vi "write_tag_status.vi"(5 "Inicio pasada":timestamp=timestamp(3789638435.424 s since 1904-01-01), 8 "Tabla_flota":string[][](array[string])=[["Flota", "UT", "Ejes", "Tag inicio", "Tag fin"], ["Prueba", "1", "4", "A0000000000000000TESTNEM7", "A0000000000000000TESTNEM8"], ["Riyadh Metro L3", "Train01", "8", "200917000000000000001196", "200917000000000000001195"], ["Riyadh Metro L3", "Train02", "8", "200917000000000000001277", "200917000000000000001293"], ["Riyadh Metro L3", "Train03", "8", "2009170000000000000012B7", "200917000000000000001259"], ["Riyadh Metro L3", "Train04", "8", "2009170000000000000011B3", "20091700000000000000119F"], ["Riyadh Metro L3", "Train05", "8", "2009170000000000000012E6", "2009170000000000000012AF"], ["Riyadh Metro L3", "Train06", "8", "200917000000000000001227", "2009170000000000000012B9"], ["Riyadh Metro L3", "Train07", "8", "200917000000000000001272", "2009170000000000000011FA"], ["Riyadh Metro L3", "Train08", "8", "200917000000000000001225", "2009170000000000000012BC"], ["Riyadh Metro L3", "Train09", "8", "200917000000000000001226", "2009170000000000000011C8"], ["Riyadh Metro L3", "Train10", "8", "2009170000000000000011FC", "2009170000000000000012B8"], ["Riyadh Metro L3", "Train11", "8", "200917000000000000001197", "20091700000000000000124C"], ["Riyadh Metro L3", "Train12", "8", "20091700000000000000124F", "2009170000000000000011BF"], ["Riyadh Metro L3", "Train13", "8", "2009170000000000000011CA", "200917000000000000001198"], ["Riyadh Metro L3", "Train14", "8", "2009170000000000000011DA", "2009170000000000000011D9"], ["Riyadh Metro L3", "Train15", "8", "20091700000000000000121C", "20091700000000000000122C"], ["Riyadh Metro L3", "Train16", "8", "2009170000000000000011B9", "200917000000000000001214"], ["Riyadh Metro L3", "Train17", "8", "200917000000000000001222", "2009170000000000000011B6"], ["Riyadh Metro L3", "Train18", "8", "200917000000000000001229", "200917000000000000001200"], ["Riyadh Metro L3", "Train19", "8", "200917000000000000001217", "200917000000000000001232"], ["Riyadh Metro L3", "Train20", "8", "2009170000000000000012B4", "2009170000000000000011CE"], ["Riyadh Metro L3", "Train21", "8", "2009170000000000000011A8", "2009170000000000000011F6"], ["Riyadh Metro L3", "Train22", "8", "200917000000000000001220", "2009170000000000000011C4"], ["Riyadh Metro L3", "Train23", "8", "2009170000000000000011EA", "200917000000000000001208"], ["Riyadh Metro L3", "Train24", "8", "200917000000000000001219", "20091700000000000000121A"], ["Riyadh Metro L3", "Train25", "8", "200917000000000000001348", "2009170000000000000012B2"], ["Riyadh Metro L3", "Train26", "8", "2009170000000000000011BD", "2009170000000000000011F7"], ["Riyadh Metro L3", "Train27", "8", "200917000000000000001207", "200917000000000000001206"], ["Riyadh Metro L3", "Train28", "8", "200917000000000000001230", "200917000000000000001322"], ["Riyadh Metro L3", "Train29", "8", "2009170000000000000011BE", "20091700000000000000124B"], ["Riyadh Metro L3", "Train30", "8", "2009170000000000000011E2", "2009170000000000000011A7"], ["Riyadh Metro L3", "Train31", "8", "2009170000000000000012BE", "2009170000000000000012BD"], ["Riyadh Metro L3", "Train32", "8", "2009170000000000000012B6", "200917000000000000001323"], ["Riyadh Metro L3", "Train33", "8", "200917000000000000001216", "20091700000000000000122A"], ["Riyadh Metro L3", "Train34", "8", "200917000000000000001274", "200917000000000000001291"], ["Riyadh Metro L3", "Train35", "8", "2009170000000000000012C4", "200917000000000000001253"], ["Riyadh Metro L3", "Train36", "8", "2009170000000000000011BC", "200917000000000000001228"], ["Riyadh Metro L3", "Train37", "8", "200917000000000000001205", "200917000000000000001292"], ["Riyadh Metro L3", "Train38", "8", "2009170000000000000011FF", "2009170000000000000011AA"], ["Riyadh Metro L3", "Train39", "8", "2009170000000000000012C5", "200917000000000000001223"], ["Riyadh Metro L3", "Train40", "8", "200917000000000000001231", "200917000000000000001199"], ["Riyadh Metro L3", "Train41", "8", "2009170000000000000011C7", "20091700000000000000121F"], ["Riyadh Metro L3", "Train42", "8", "2009170000000000000011AC", "2009170000000000000011AB"], ["Riyadh Metro L3", "Train43", "8", "20091700000000000000121D", "200917000000000000001302"], ["Riyadh Metro L3", "Train44", "8", "2009170000000000000011CD", "2009170000000000000011E1"], ["Riyadh Metro L3", "Train45", "8", "2009170000000000000012B0", "2009170000000000000011A0"], ["Riyadh Metro L3", "Train46", "8", "2009170000000000000012BB", "2009170000000000000012BA"], ["Riyadh Metro L3", "Train47", "8", "20091700000000000000119C", "20091700000000000000119B"]], 9 "TagData in":cluster{"TagCode":string, "FirstSeemUs":u64}[](array[cluster]), 10 "file path (use dialog)":path=path "c:/RFID/status.csv") -> ()   [LabVIEW 2015]
panel:
  out "Fin":i32
  out "Ini":i32
  out "size(s)":i32
  out "Tag Fin":string="0"
  out "Tag Ini":string="0"
  out "s? t:f":i32
  out "substring":string
  in  "Train":string="Train01"
  out "Text":string
  out "concatenated string":string
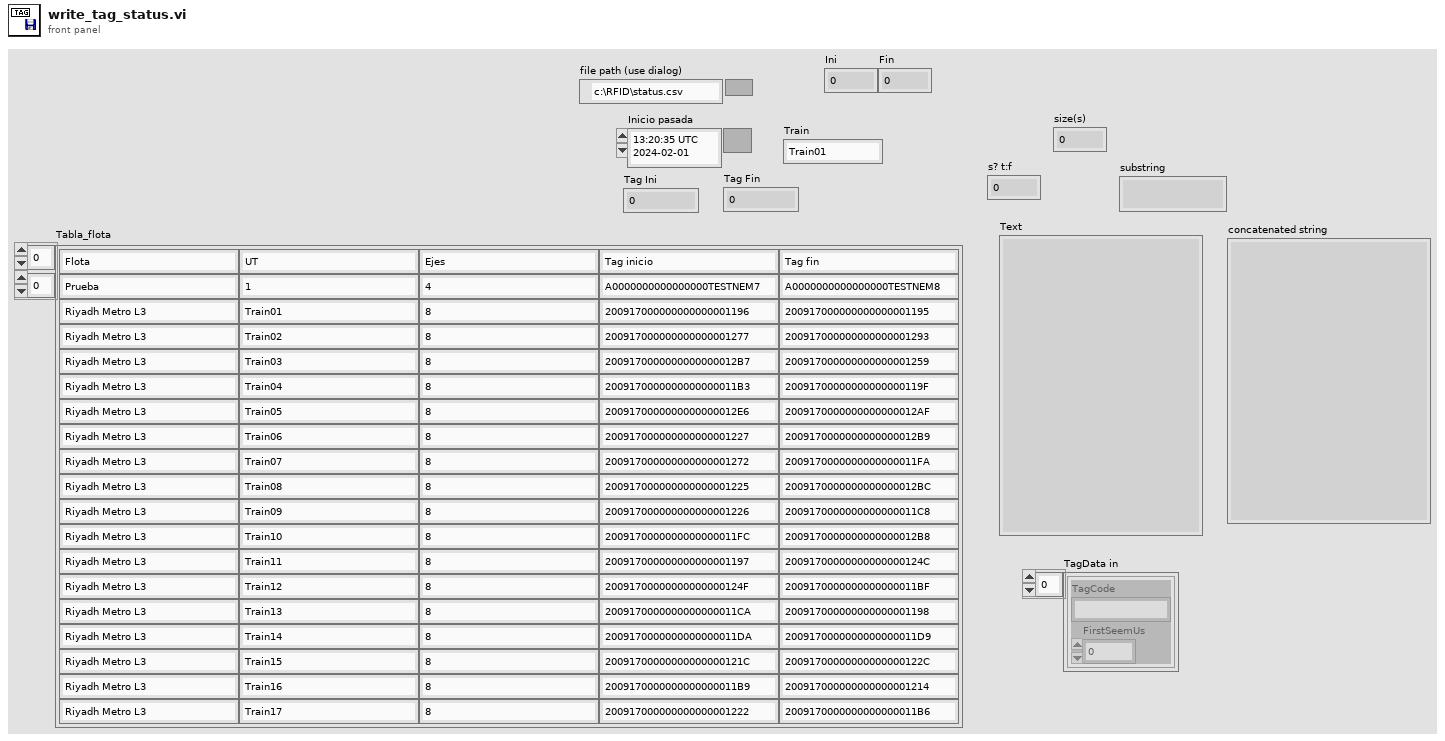
[diagram p1: front panel]
types:
  T1 = enum16{"open", "replace", "create", "open or create", "replace or create", "replace or create with confirmation"}
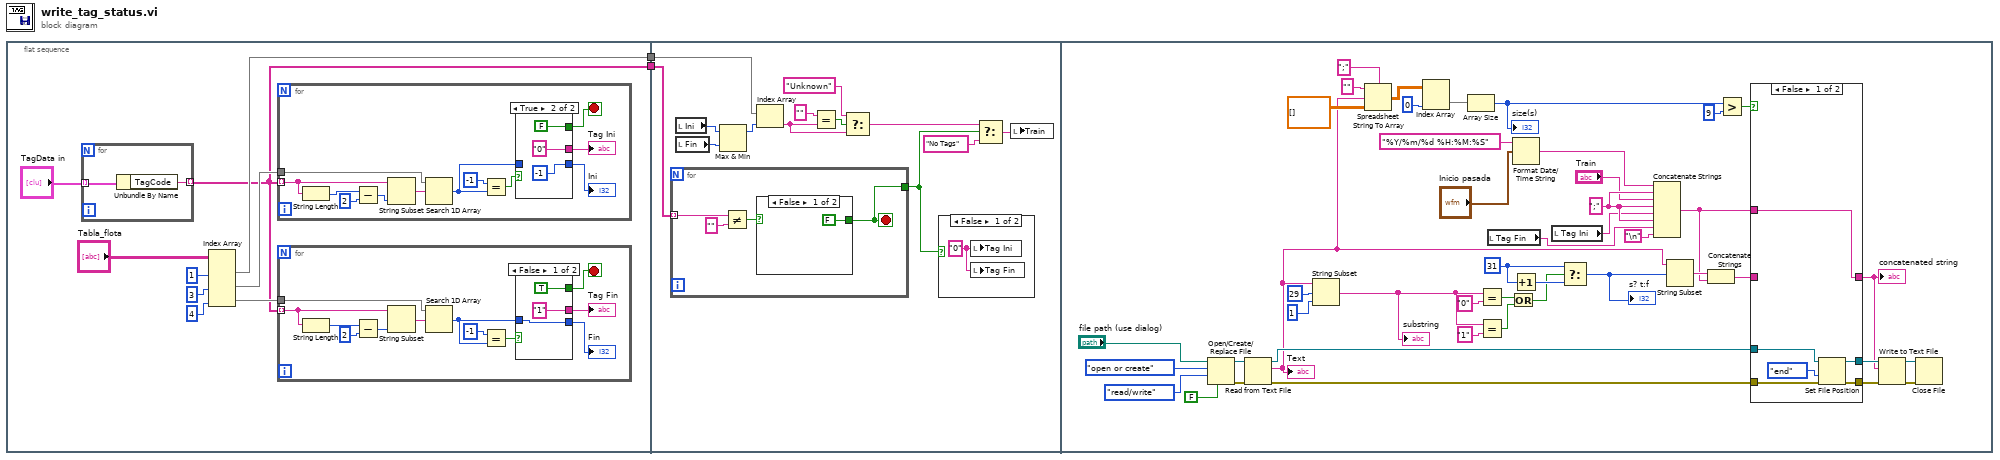
[diagram p0: block diagram]
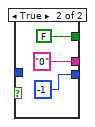
[diagram p2: hidden frame]
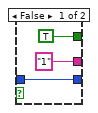
[diagram p3: hidden frame]
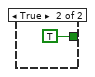
[diagram p5: hidden frame]
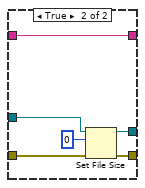
[diagram p6: hidden frame]
diagram:
  n1 = flat-sequence {
    tunnel: [w5] -> w2
    tunnel: [w4] -> w1
    tunnel: w2 -> [w52]
    tunnel: w1 -> [w51]
    frame #0 {
      n2 = for {
        tunnel: "TagData in" -> [w49] mode=indexing
        tunnel: [w48] -> w4 mode=indexing
        n3 = Unbundle By Name(w49) -> ("TagCode"=w48:string)
      }
      n4 = Index Array(array="Tabla_flota", index (col) #1=1 ("index (row)"), index (col) #2=3 ("disabled index (col)"), index (col) #3=4 ("disabled index (col)")) -> (element #1=w5:string[], element #2=w10:string[], element #3=w11:string[])  [unwired: 3 in]
      n5 = for {
        tunnel: w4 -> [w38] mode=indexing
        tunnel: w10 -> [w41]
        stop <- w33 stop-if-true
        n6 = String Length(string=w38) -> (length=w35:i32)
        n7 = Subtract(x=w35, y=2) -> (x-y=w36:i32)
        n8 = String Subset(string=w38, length (rest)=w36) -> (substring=w37:string)  [unwired: 1 in]
        n9 = Search 1D Array(1D array=w41, element=w37) -> (index of element=w31:i32)  [unwired: 1 in]
        n10 = Equal?(x=-1, y=w31) -> (x = y?=w39:bool)
        n11 = case shown="True" w39 {
          tunnel: ["1" ("Tag Ini") "0" ("Tag Ini")] -> w32
          tunnel: [TRUE FALSE] -> w33
          tunnel: w31 -> [w42 _]
          tunnel: [w42 -1 ("x")] -> w30
          frame False {
          }
          frame True {
          }
        }
        "Tag Ini" <- w32
        "Ini" <- w30
      }
      n12 = for {
        tunnel: w4 -> [w20] mode=indexing
        tunnel: w11 -> [w23]
        stop <- w15 stop-if-true
        n13 = String Length(string=w20) -> (length=w17:i32)
        n14 = Subtract(x=w17, y=2) -> (x-y=w18:i32)
        n15 = String Subset(string=w20, length (rest)=w18) -> (substring=w19:string)  [unwired: 1 in]
        n16 = Search 1D Array(1D array=w23, element=w19) -> (index of element=w13:i32)  [unwired: 1 in]
        n17 = Equal?(x=-1, y=w13) -> (x = y?=w21:bool)
        n18 = case shown="False" w21 {
          tunnel: ["1" ("Tag Ini") "0" ("Tag Ini")] -> w14
          tunnel: [TRUE FALSE] -> w15
          tunnel: w13 -> [w24 _]
          tunnel: [w24 -1 ("x")] -> w12
          frame False {
          }
          frame True {
          }
        }
        "Tag Fin" <- w14
        "Fin" <- w12
      }
    }
    frame #1 {
      n19 = for {
        tunnel: w51 -> [w67] mode=indexing
        tunnel: [w64] -> w50
        stop <- w64 stop-if-true
        n20 = Not Equal?(x=w67, y="") -> (x != y?=w65:bool)
        n21 = case shown="False" w65 {
          tunnel: [FALSE TRUE] -> w64
          frame False {
          }
          frame True {
          }
        }
      }
      n22 = local read "Ini"() -> (w54:i32)
      n23 = local read "Fin"() -> (w56:i32)
      n24 = Max & Min(x=w54, y=w56) -> (max(x,y)=w62:i32)  [unwired: 1 out]
      n25 = Index Array(array=w52, index=w62) -> (element=w58:string)
      n26 = Equal?(x="" ("y"), y=w58) -> (x = y?=w61:bool)
      n27 = Select(t="Unknown", s=w61, f=w58) -> (s? t:f=w55:string)
      n28 = case shown="False" w50 {
        frame False {
          w63 = "0" ("Tag Ini")
          n29 = local write "Tag Ini"(w63) -> ()
          n30 = local write "Tag Fin"(w63) -> ()
        }
        frame True {
        }
      }
      n31 = Select(t=w55, s=w50, f="No Tags") -> (s? t:f=w57:string)
      n32 = local write "Train"(w57) -> ()
    }
    frame #2 {
      w79 = 31 ("offset (0)")
      w82 = ";" ("string")
      n33 = Open/Create/Replace File(file path (use dialog)="file path (use dialog)", operation (0:open)=T1."open or create", access (0:read/write)=enum16{"read/write", "read-only", "write-only"}."read/write", disable buffering (F)=FALSE) -> (refnum out=w105:refnum<file>, error out=w104:errorcluster)  [unwired: 1 in, 2 out]
      n34 = Read from Text File(file (use dialog)=w105, error in=w104) -> (refnum out=w103:refnum<file>, text=w88:string, error out=w102:errorcluster)  [unwired: 2 in, 1 out]
      "Text" <- w88
      n35 = String Subset(string=w88, offset (0)=29, length (rest)=1 ("length (rest)")) -> (substring=w74:string)
      "substring" <- w74
      n36 = Spreadsheet String To Array(delimiter (Tab)=";", format string="", spreadsheet string=w88, array type (2D Dbl)=dbl[][] []) -> (array=w98:dbl[][])
      n37 = Index Array(array=w98, index (col)=0 ("index (row)")) -> (element=w97:dbl[])  [unwired: 1 in]
      n38 = Array Size(array=w97) -> (size(s)=w95:i32)
      "size(s)" <- w95
      n39 = Equal?(x=w74, y="0") -> (x = y?=w77:bool)
      n40 = Equal?(x=w74, y="1") -> (x = y?=w76:bool)
      n41 = local read "Tag Fin"() -> (w70:string)
      n42 = Or(x=w77, y=w76) -> (x .or. y?=w78:bool)
      n43 = Format Date/Time String(time format string (%c)="%Y/%m/%d %H:%M:%S", seconds (now)="Inicio pasada") -> (date/time string=w110:string)  [unwired: 1 in]
      n44 = Increment(x=w79) -> (x+1=w91:i32)
      n45 = local read "Tag Ini"() -> (w71:string)
      n46 = Select(t=w79, s=w78, f=w91) -> (s? t:f=w90:i32)
      "s? t:f" <- w90
      n47 = Concatenate Strings(w110, w82, "Train", w82, w71, w82, w70, "\n") -> (w84:string)
      n48 = String Subset(string=w88, offset (0)=w90) -> (substring=w87:string)  [unwired: 1 in]
      n49 = Concatenate Strings(w87, w84) -> (w85:string)
      n50 = Greater?(x=w95, y=9) -> (0:w86:bool)
      n51 = case shown="False" w86 {
        tunnel: [w119 w123] -> w107
        tunnel: [w118 w124] -> w106
        tunnel: w103 -> [w117 w125]
        tunnel: w102 -> [w116 w122]
        tunnel: [w115 w126] -> w83
        tunnel: w85 -> [_ w126]
        tunnel: w84 -> [w115 _]
        frame False {
          n52 = Set File Position(refnum=w117, from (0:start)=enum16{"start", "end", "current"}."end", error in=w116) -> (refnum out=w118:refnum<file>, error out=w119:errorcluster)  [unwired: 1 in]
        }
        frame True {
          n53 = Set File Size(4:w122, 6:i64 0 ("size (in bytes)"), 7:w125) -> (0:w123:errorcluster, 3:w124:refnum<file>)
        }
      }
      "concatenated string" <- w83
      n54 = Write to Text File(file (use dialog)=w106, text=w83, error in=w107) -> (refnum out=w109:refnum<file>, error out=w108:errorcluster)  [unwired: 1 in, 1 out]
      n55 = Close File(refnum=w109, error in=w108) -> ()  [unwired: 2 out]
    }
  }
